vi "GUI_HTU_Chicane.vi"() -> ()   [LabVIEW 2013]
uses:
  Shared/GUI_Template/GUI_master/tcp_new_data_event.ctl
  Shared/GUI_Template/GUI_master/tcp new data cluster.ctl
panel:
  in  "Voltage::1":dbl caption="Outer Voltage" min=0.0 max=15.0
  in  "Voltage::2":dbl caption="Inner Voltage" min=0.0 max=15.0
  in  "Enable_Output::2":enum16{"on", "off"}(ring) caption="Enable output inner"
  in  "Enable_Output::1":enum16{"on", "off"}(ring) caption="Enable output outer"
  in  "RunList::2":enum16{"on", "off"}(ring) caption="Run List Inner Pair"
  in  "RunList::1":enum16{"on", "off"}(ring) caption="Run List Outer Pair"
  in  "LoadList::2":enum16{"on", "off"}(ring) caption="Load List Inner Pair"
  in  "LoadList::1":enum16{"on", "off"}(ring) caption="Load List Outer Pair"
  out "Chart":dbl[][](graph)
  in  "ApplyChicaneSettings":bool
  in  "Energy (MeV)":dbl=100.0
  in  "R56 (microns)":dbl
  out "Offset (mm)":dbl
  out "Width of 2% \nenergy spread (mm)":dbl
  out "SetCurrent":dbl
  in  "CalculateChicaneSettings":bool
  in  "Current::1":dbl caption="Outer Current" min=-12.0 max=12.0
  in  "Current::2":dbl caption="Inner Current" min=-12.0 max=12.0
  out "error IO 2":errorcluster
  out "tcp data event":T1
  in  "UDP error message":string
  in  "GUIdevice 2":string="U_ChicaneInner"
  in  "GUIdevice 1":string="U_ChicaneOuter"
  in  "stop":bool
  # "HTU Chicane"
  # "Energy"
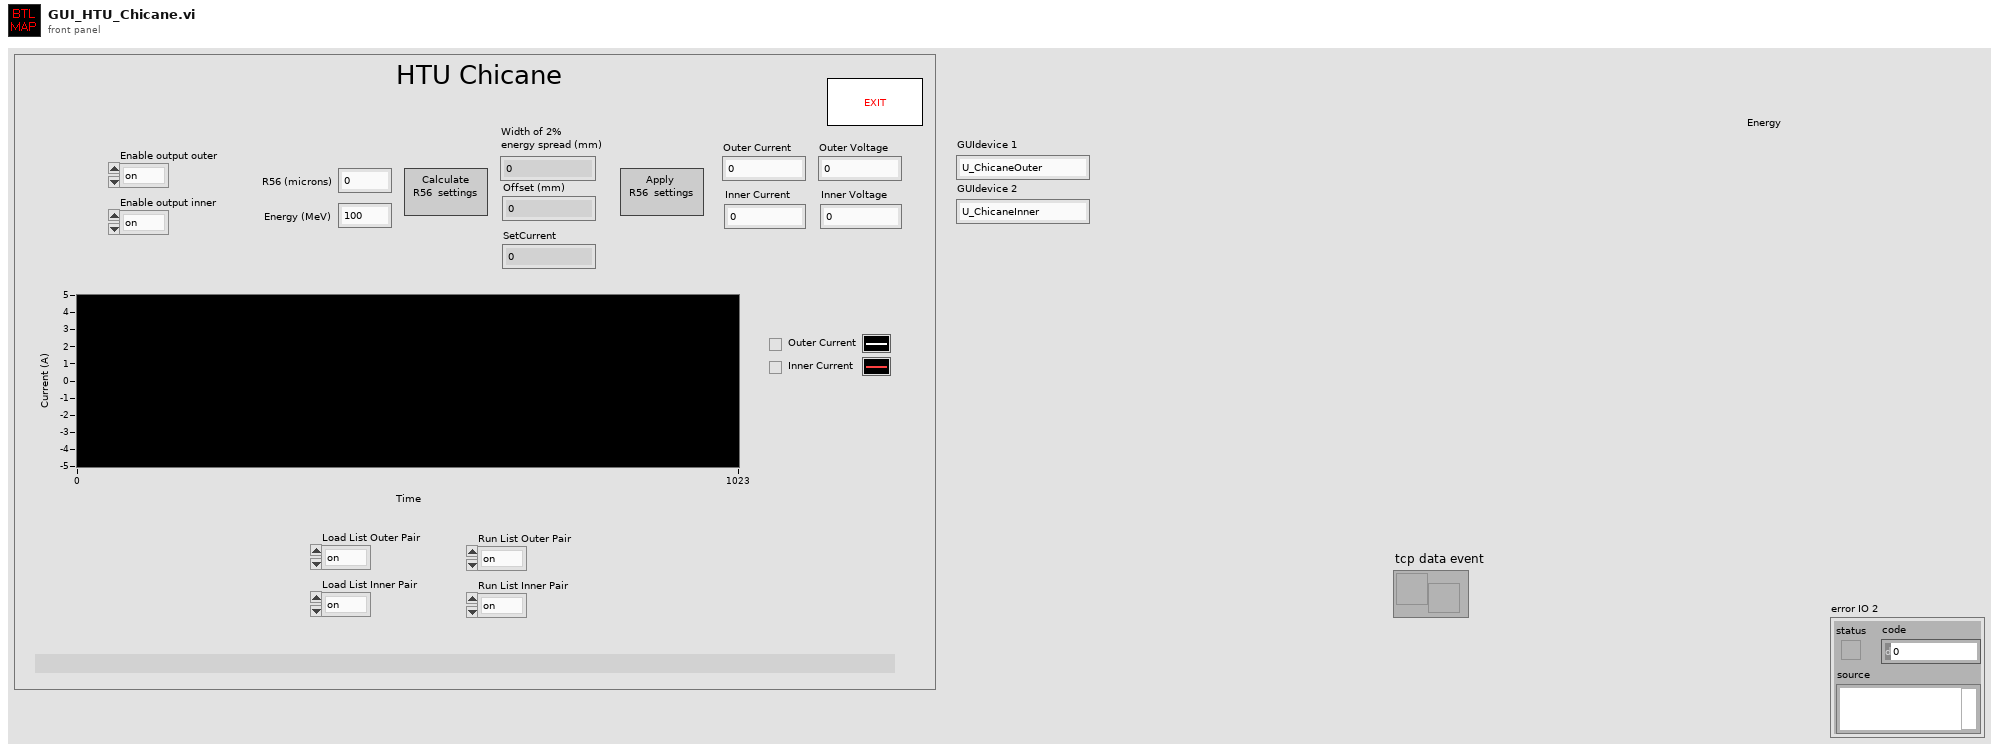
[diagram p1: front panel]
types:
  T1 = typedef "tcp_new_data_event.ctl" = refnum<user-event>
  T2 = typedef "tcp new data cluster.ctl" = cluster{"EventEnum":enum16{"new data", "connection status update"}, "Device name":string}
  T3 = enum32{"invalid app kind", "Development System", "Run Time System", "Student Edition", "Embedded LabVIEW", "Evaluation", "Custom"}
  T4 = enum32{"Invalid", "Standard", "Closed", "Hidden", "Minimized", "Maximized"}
  T5 = cluster{"Core":cluster{"Current VI Reference":refnum<vi>, "Close Panel on Exit?":bool}, "CalculateChicanceSettings":bool, "ApplyChicanceSettings":bool, "CurrentGraph1":dbl[][], "CurrentGraph2":dbl[][]}
  T6 = cluster{"Current VI Reference":refnum<vi>, "Close Panel on Exit?":bool}
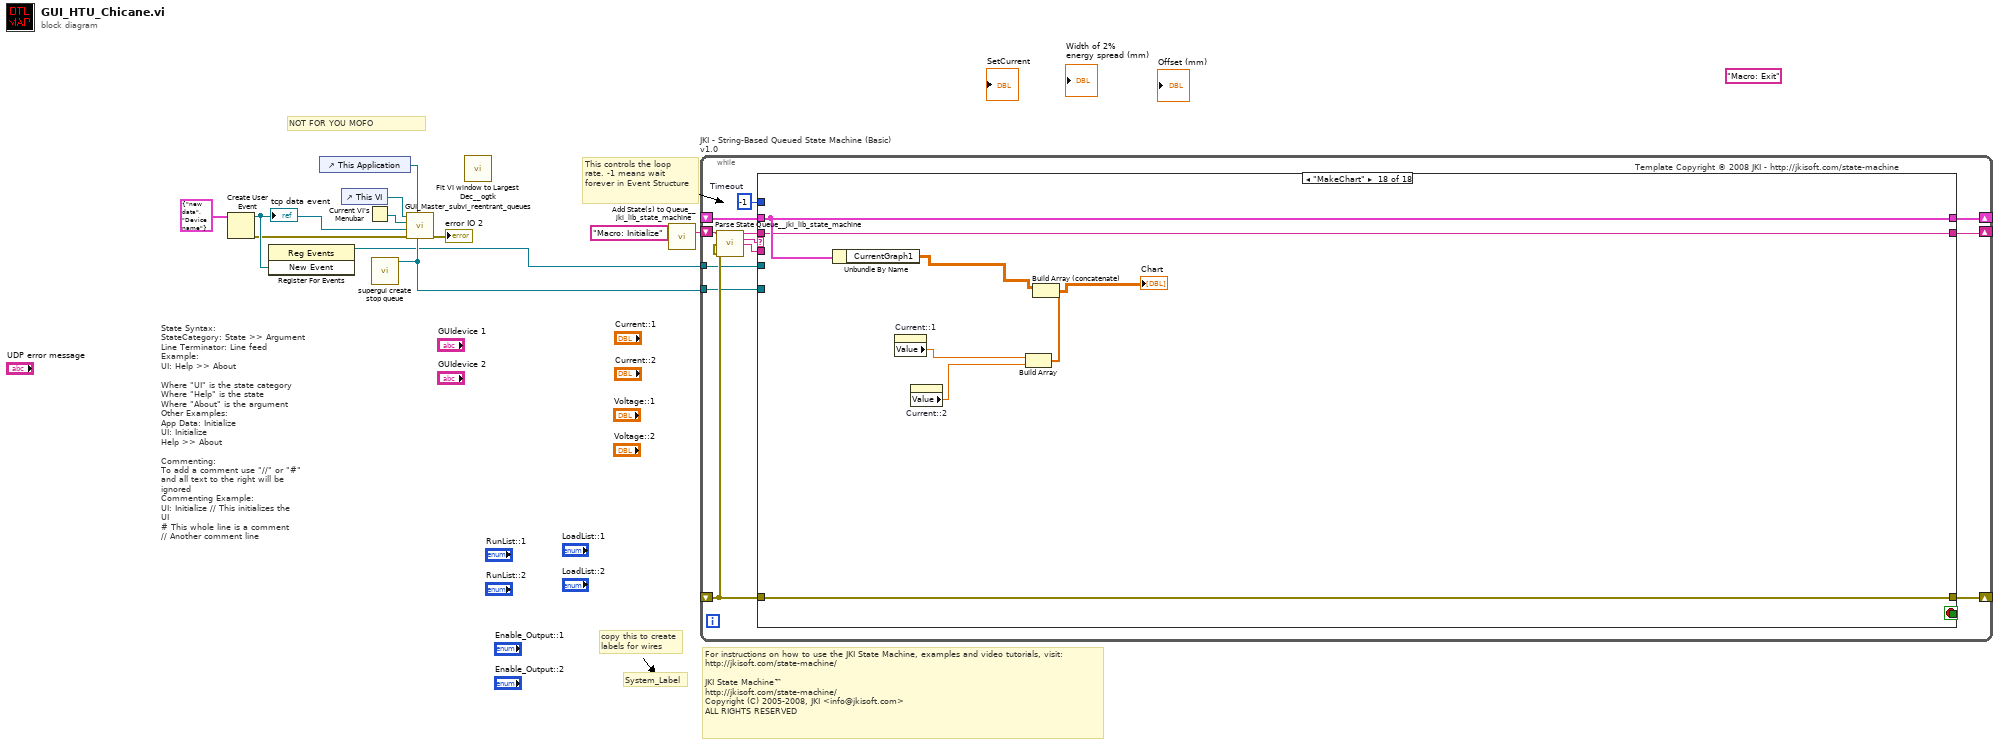
[diagram p0: block diagram]
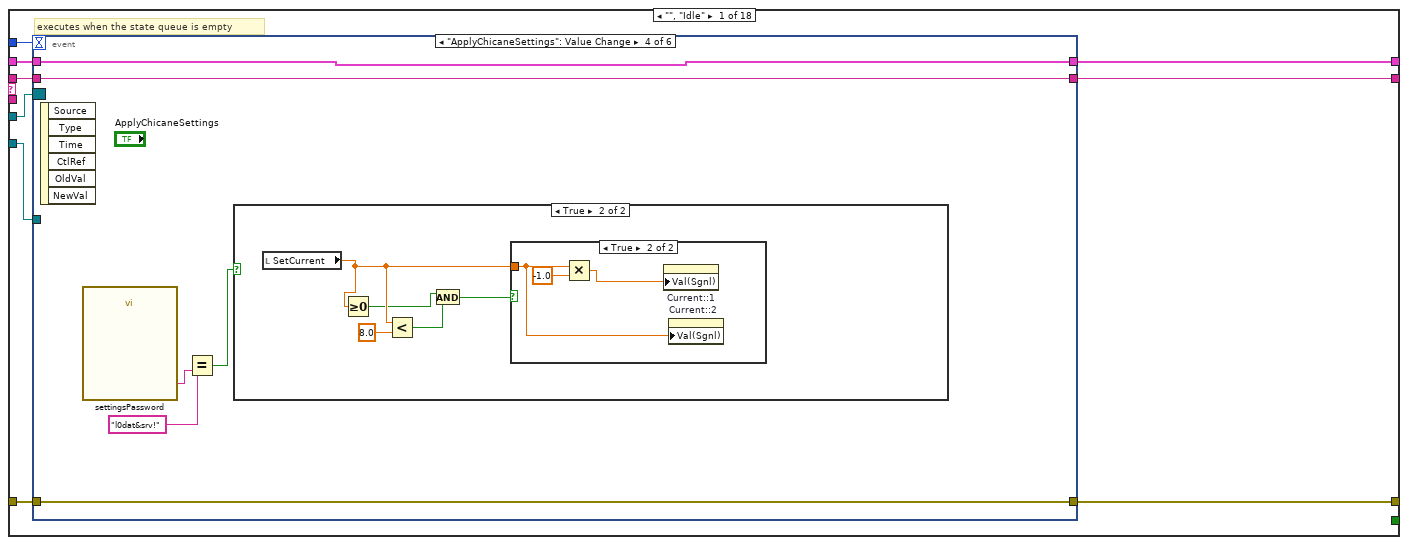
[diagram p2: hidden frame]
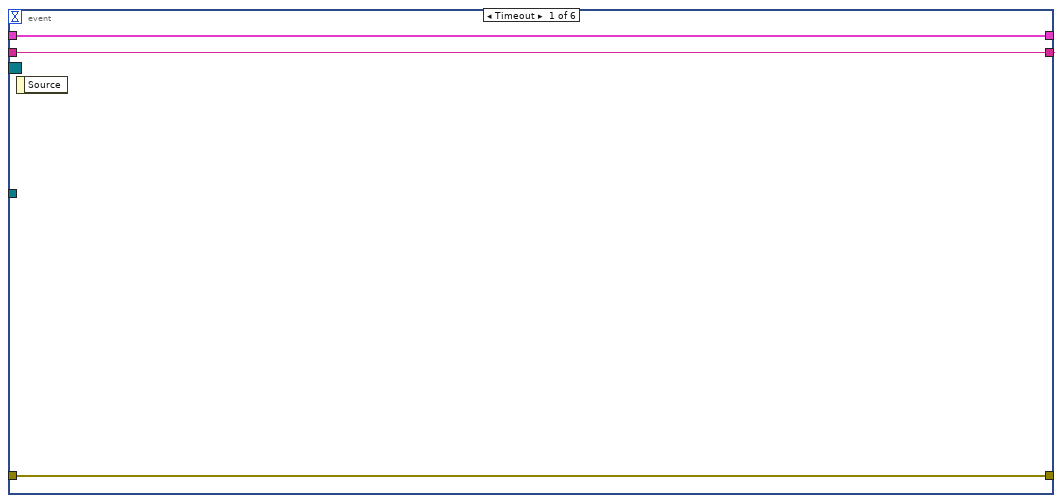
[diagram p3: hidden frame]
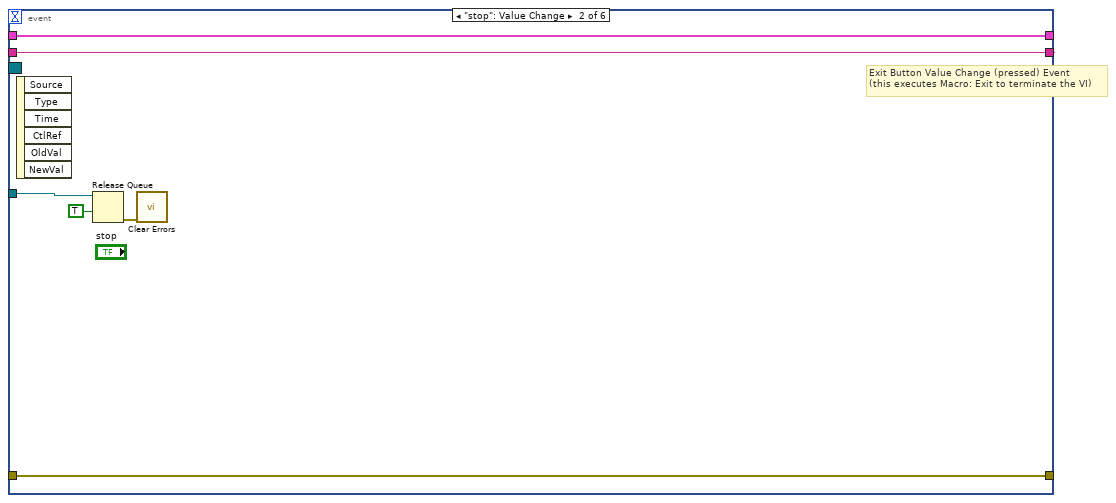
[diagram p4: hidden frame]
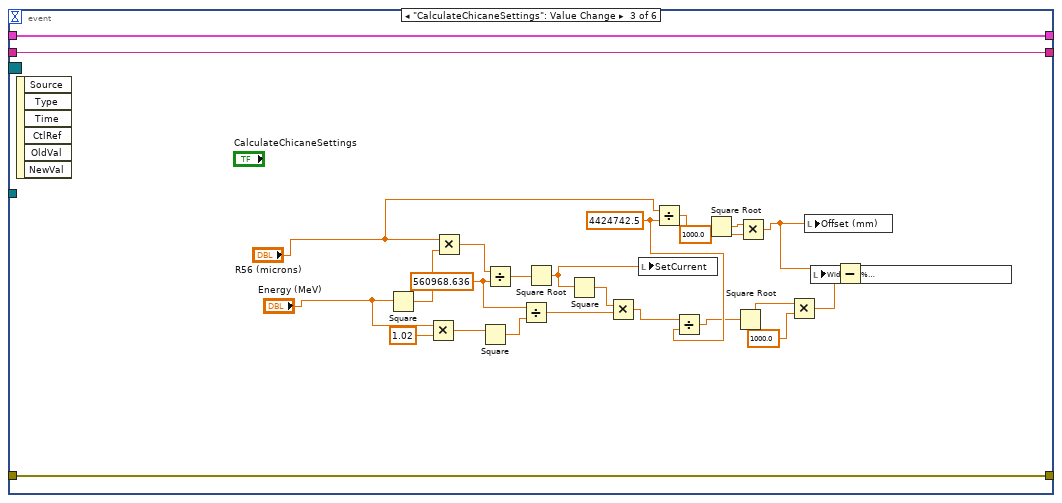
[diagram p5: hidden frame]
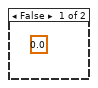
[diagram p6: hidden frame]
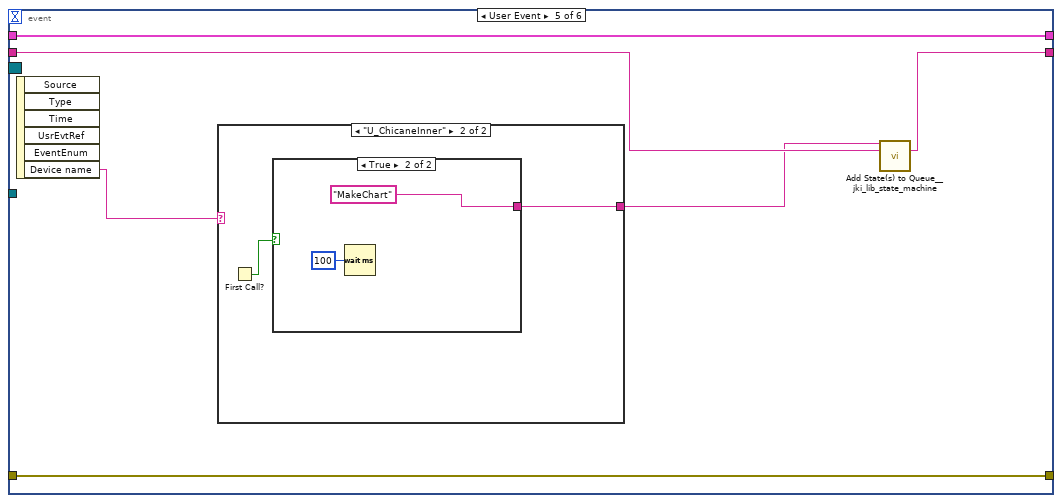
[diagram p8: hidden frame]
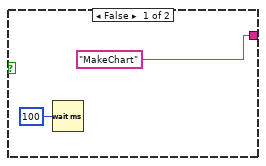
[diagram p10: hidden frame]
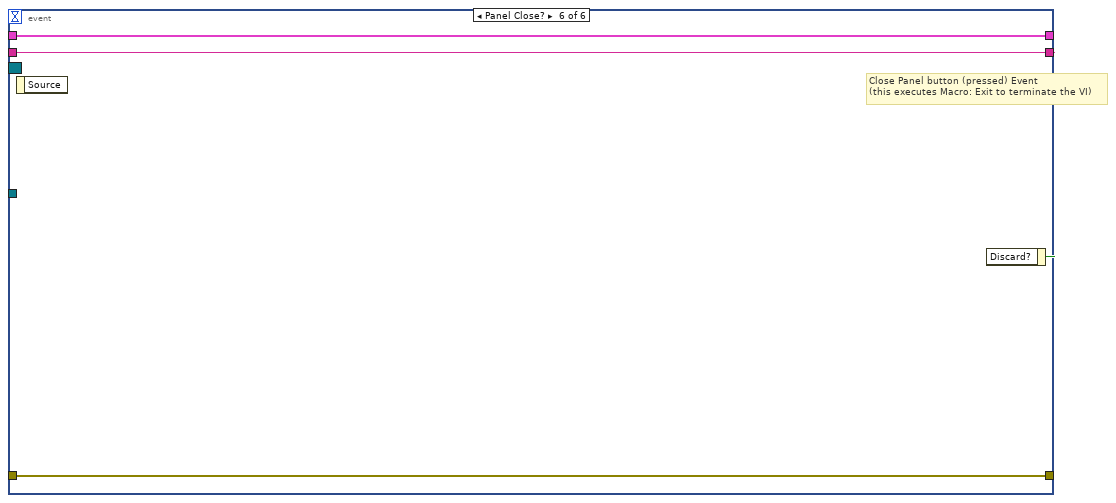
[diagram p11: hidden frame]
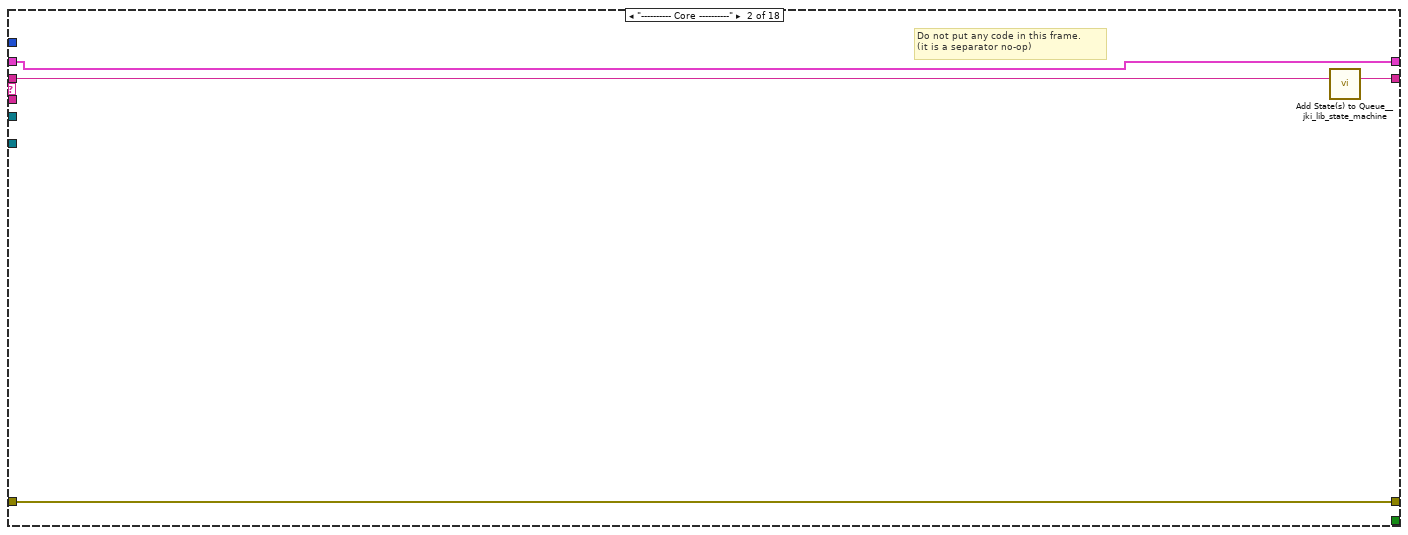
[diagram p12: hidden frame]
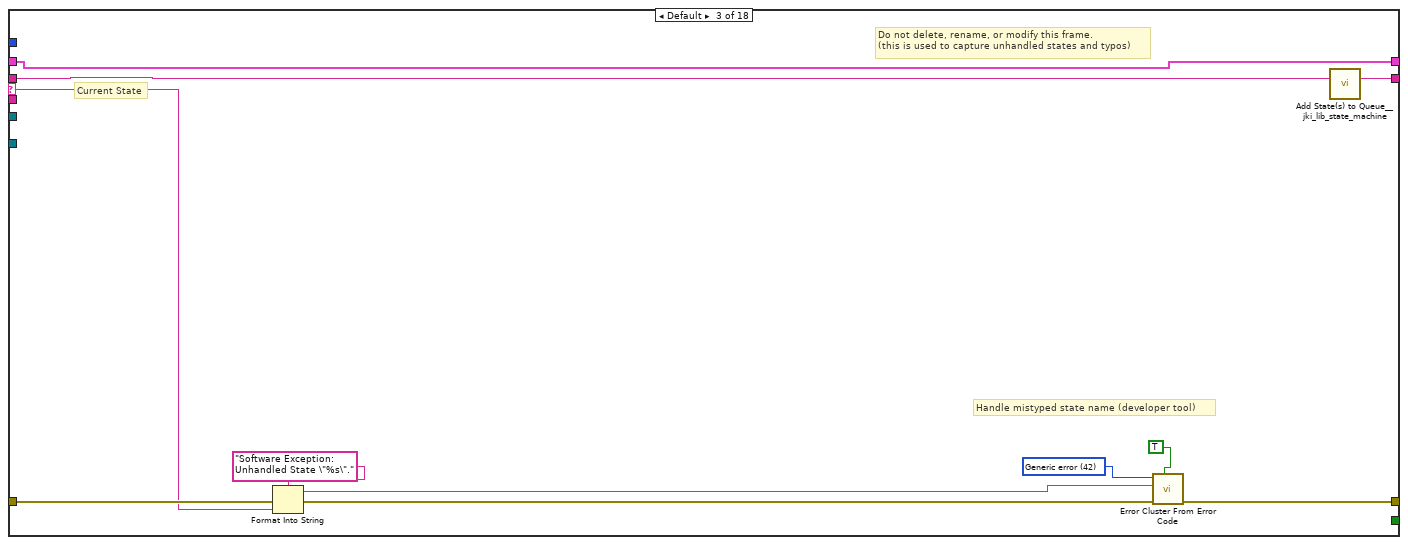
[diagram p13: hidden frame]
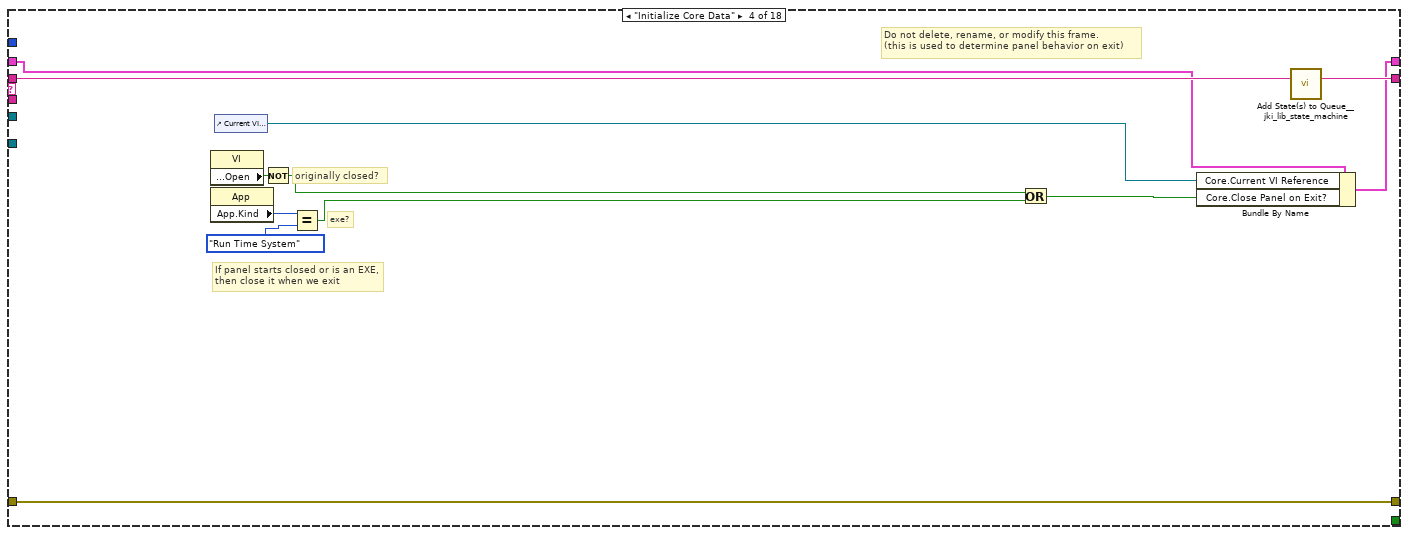
[diagram p14: hidden frame]
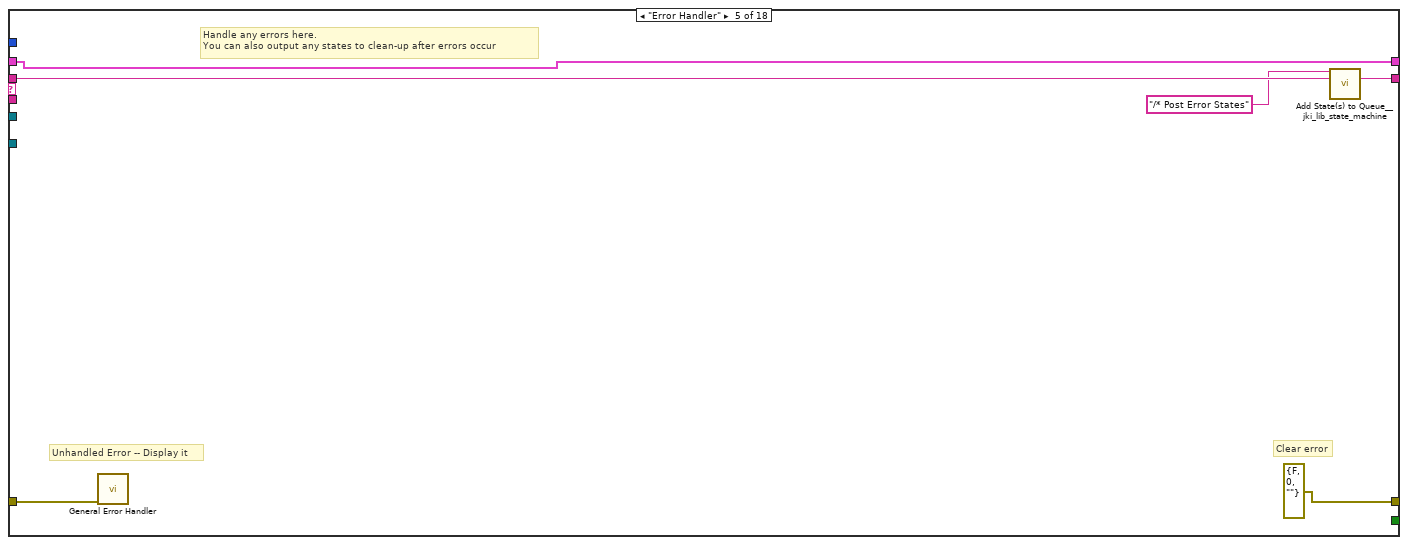
[diagram p15: hidden frame]
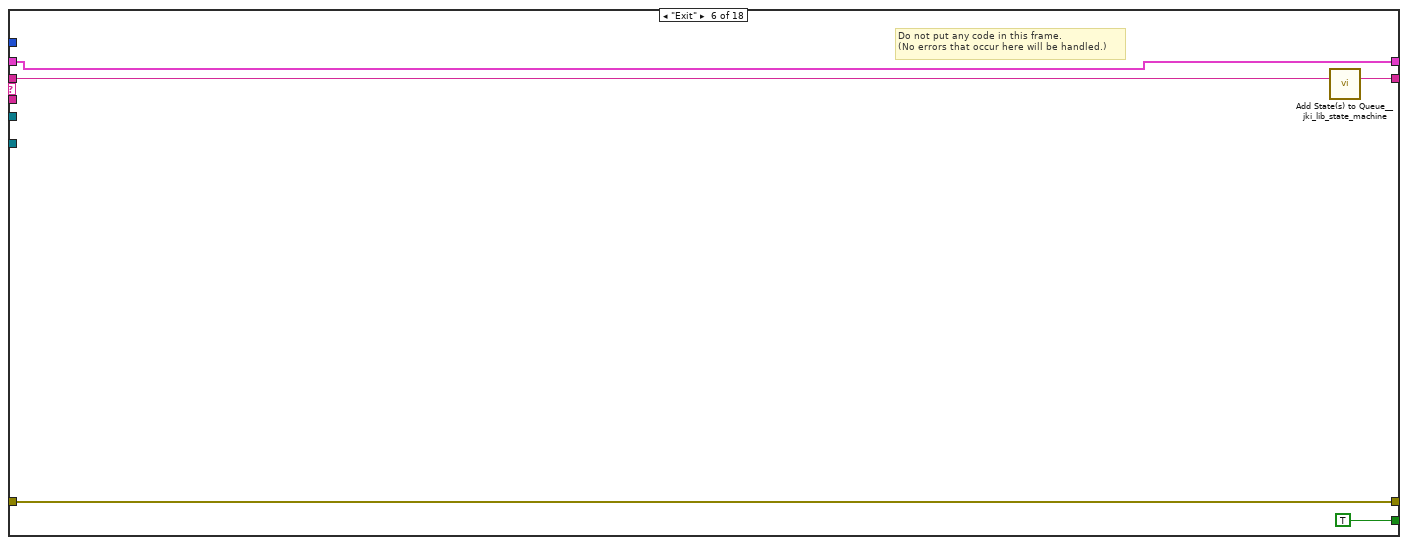
[diagram p16: hidden frame]
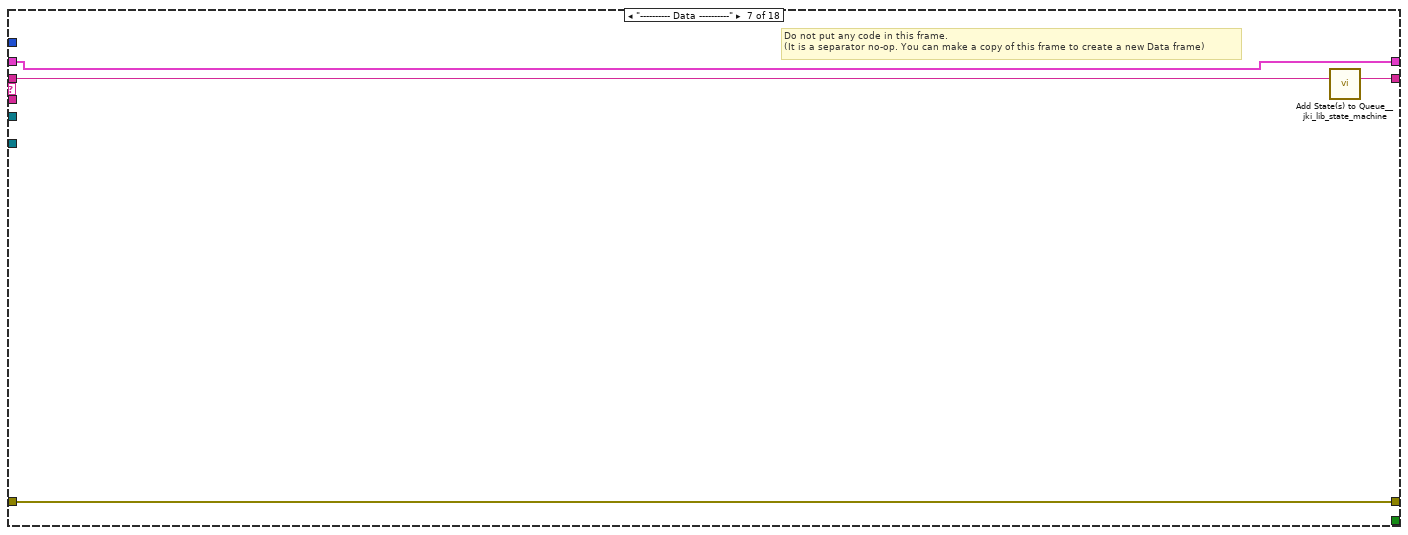
[diagram p17: hidden frame]
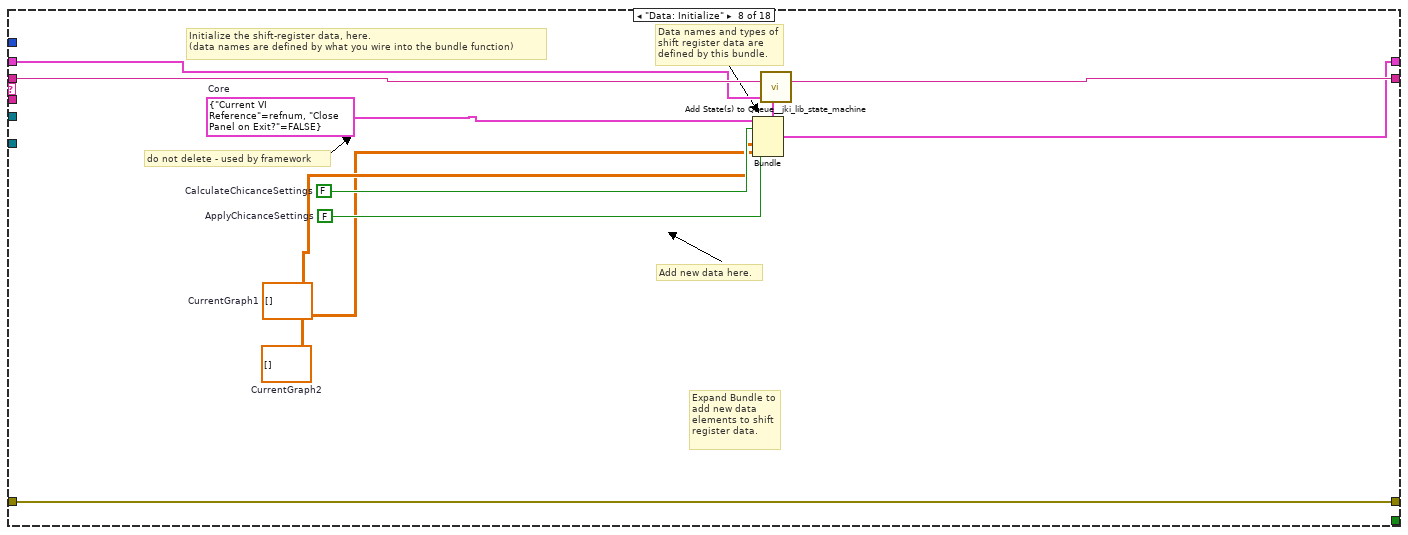
[diagram p18: hidden frame]
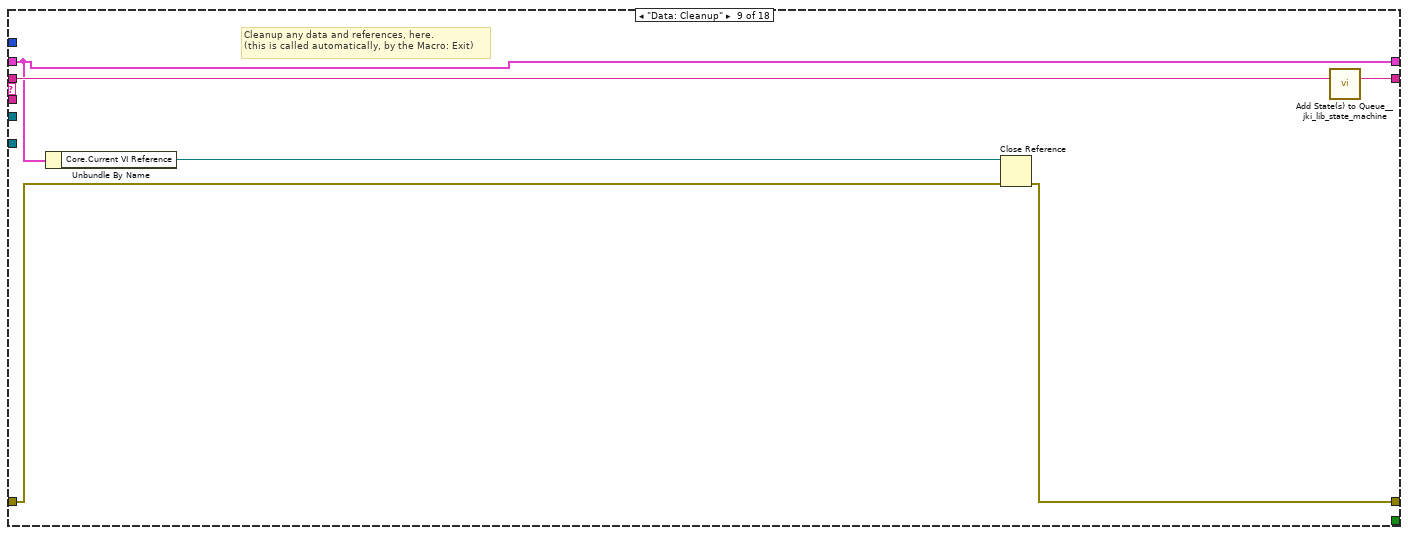
[diagram p19: hidden frame]
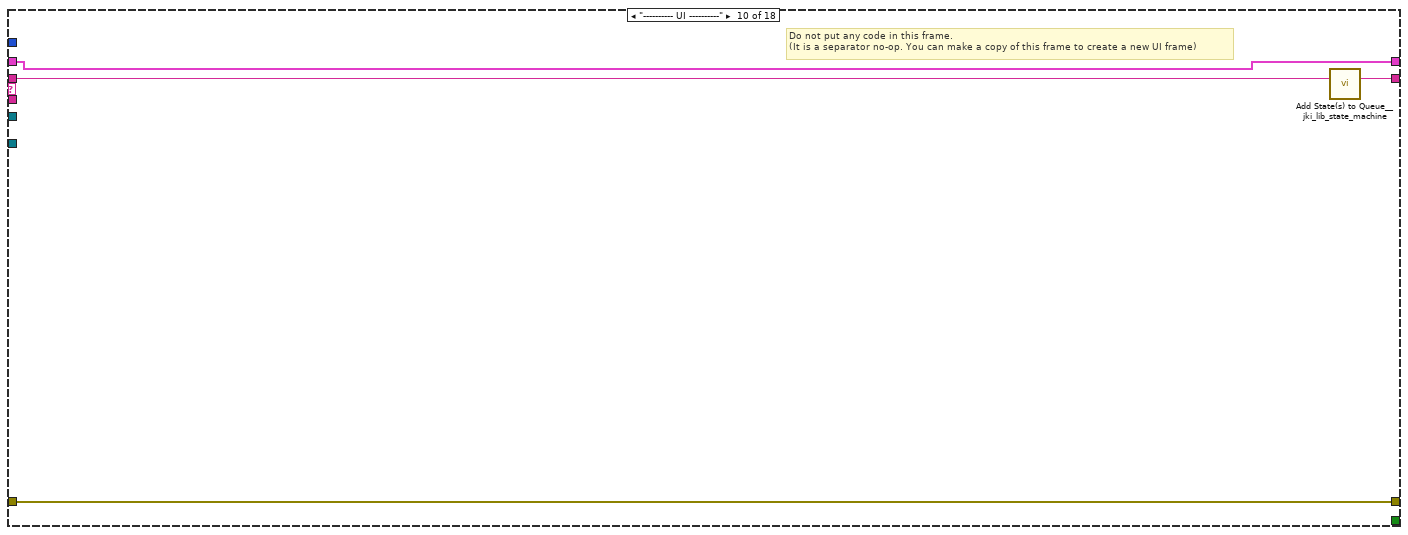
[diagram p20: hidden frame]
diagram:
  (unwired) "Macro: Exit"
  # "For instructions on how to use the JKI State Machine, examples and video tutorials, visit:\nhttp://jkisoft.com/state-machine/\n\nJKI State Machine™\nhttp://jkisoft.com/state-machine/\nCopyright (C) 2005-2008, JKI <info@jkisoft.com>\nALL RIGHTS RESERVED"
  # "State Syntax:\nStateCategory: State >> Argument\nLine Terminator: Line feed\nExample:\nUI: Help >> About\n\nWhere \"UI\" is the state category\nWhere \"Help\" is the state\nWhere \"About\" is the argument\nOther Examples:\nApp Data: Initialize\nUI: Initialize\nHelp >> About\n\nCommenting:\nTo add a comment use \"//\" or \"#\" and all text to the right will be ignored\nCommenting Example:\nUI: Initialize // This initializes the UI\n# This whole line is a comment\n// Another comment line"
  # "copy this to create labels for wires"
  # "This controls the loop rate. -1 means wait forever in Event Structure"
  # "System_Label"
  # "NOT FOR YOU MOFO"
  n1 = Create User Event(user event datatype=T2 {"EventEnum"=enum."new data", "Device name"="Device name"} ("New Event")) -> (user event=w10:refnum<user-event>, error out=w9:errorcluster)  [unwired: 1 in]
  "tcp data event" <- w10
  n2 = register-events(w10) -> (reference out=w1:refnum<event-registration>)  [unwired: 2 in, 1 out]
  n3 = control-ref of="This Application"() -> (w11:refnum<vi>)
  n4 = control-ref of="This VI"() -> (w5:refnum<vi>)
  n5 = Current VI's Menubar() -> (w7:refnum<k9>)
  n6 = call "supergui create stop queue.vi"() -> ("STOP Queue out"=w2:refnum<queue>)  [unwired: 11 in]
  n7 = call "GUI_Master_subvi_reentrant_queues.vi"("STOP Queue in"=w2, "This Application"=w11, "error in (no error)"=w9, "tcp data event"=w10, "Caller menu reference"=w7, "Caller VI ref"=w5) -> ("error out"=→"error IO 2":errorcluster)  [unwired: 5 in]
  n8 = call <userlib>:"Fit VI window to Largest Dec__ogtk.vi"() -> ()  [unwired: 6 in, 2 out]
  n9 = call <vilib>:"Add State(s) to Queue__jki_lib_state_machine.vi"("State(s) in (\"\")"="Macro: Initialize") -> ("States Out"=w3:string)  [unwired: 14 in]
  n10 = while "JKI - String-Based Queued State Machine (Basic) v1.0" {
    shift-right: [w17] -> _
    shift-left: _ -> [w16]
    shift-right: [w20] -> _
    shift-left: _ -> [w14]
    shift-right: [w19] -> _
    shift-left: w3 -> [w21]
    tunnel: w1 -> [w13]
    tunnel: w2 -> [w12]
    stop <- w18 stop-if-true
    w15 = -1  # Timeout
    # "Template Copyright © 2008 JKI - http://jkisoft.com/state-machine"
    n11 = call <vilib>:"Parse State Queue__jki_lib_state_machine.vi"("State Queue"=w21, "Error In (no error)"=w14) -> ("Remaining States"=w23:string, "Current State"=w24:string, "Arguments"=w22:string)  [unwired: 11 in]
    n12 = case shown="\"MakeChart\"" w24 {
      selector: w24 -> [_ _ w108 _ _ _ _ _ _ _ _ _ _ _ _ _ _ _]
      tunnel: w23 -> [w33 w107 w112 w130 w136 w141 w145 w155 w161 w165 w169 w175 w186 w212 w217 w227 w231 w236]
      tunnel: w22 -> [_ _ _ _ _ _ _ _ _ _ _ w170 w181 _ _ _ _ _]
      tunnel: w16 -> [w31 w104 w110 w120 w133 w139 w142 w150 w156 w162 w167 w173 w180 w209 w214 w218 w228 w237]
      tunnel: [w30 w105 w114 w128 errorcluster {"status"=FALSE, "code"=0, "source"=""} ("error out") w138 w143 w153 w158 w163 w166 w171 w183 w210 w215 w225 w229 w235] -> w20
      tunnel: w14 -> [w29 w105 w113 w128 w132 w138 w143 w153 w159 w163 w166 w172 w184 w210 w215 w225 w229 w235]
      tunnel: [w32 w106 w111 w129 w135 w140 w144 w154 w160 w164 w168 w174 w185 w211 w216 w226 w230 w236] -> w19
      tunnel: [_ _ _ _ _ TRUE _ _ _ _ _ _ _ _ _ _ _ _] -> w18
      tunnel: [w25 w104 w110 w119 w133 w139 w142 w149 w156 w162 w167 w173 w180 w209 w214 w218 w228 w237] -> w17
      tunnel: w15 -> [w28 _ _ _ _ _ _ _ _ _ _ _ _ _ _ _ _ _]
      tunnel: w13 -> [w27 _ _ _ _ _ _ _ _ _ _ _ _ _ _ _ _ _]
      tunnel: w12 -> [w26 _ _ _ _ _ _ _ _ _ _ _ _ _ _ _ _ _]
      frame "", "Idle" {
        # "executes when the state queue is empty"
        n13 = event shown="[3] \"ApplyChicaneSettings\": Value Change" {
          selector: w27 -> [_ _ _ _ _ _]
          dyn-events: _ -> [_ _ _ _ _ _]
          timeout: w28 -> [_ _ _ _ _ _]
          tunnel: w33 -> [w37 w45 w71 w77 w89 w103]
          tunnel: [w36 w44 w71 w77 w87 w102] -> w32
          tunnel: w31 -> [w34 w42 w69 w73 w90 w100]
          tunnel: [w35 w43 w70 w76 w86 w101] -> w30
          tunnel: w29 -> [w35 w43 w70 w76 w86 w101]
          tunnel: [w34 w42 w69 w73 w90 w100] -> w25
          tunnel: w26 -> [_ w39 _ _ _ _]
          event Timeout {
            n14 = event-data() -> ()  [unwired: 1 in, 1 out]
            n15 = call <vilib>:"Add State(s) to Queue__jki_lib_state_machine.vi"("State(s) in (\"\")"=w37) -> ("States Out"=w36:string)  [unwired: 14 in]
          }
          event "stop": Value Change {
            # "Exit Button Value Change (pressed) Event\n(this executes Macro: Exit to terminate the VI)"
            n16 = event-data() -> ()  [unwired: 1 in, 6 out]
            n17 = Release Queue(queue=w39, force destroy? (F)=TRUE) -> (error out=w40:errorcluster)  [unwired: 1 in, 2 out]
            n18 = call <vilib>:"Clear Errors.vi"("error in (no error)"=w40) -> ()  [unwired: 6 in, 1 out]
            n19 = call <vilib>:"Add State(s) to Queue__jki_lib_state_machine.vi"("State(s) in Front (\"\")"="Macro: Exit", "State(s) in (\"\")"=w45) -> ("States Out"=w44:string)  [unwired: 13 in]
          }
          event "CalculateChicaneSettings": Value Change {
            w52 = 4424742.5 ("y")
            w59 = 560968.636 ("y")
            n20 = event-data() -> ()  [unwired: 1 in, 6 out]
            n21 = Square(x="Energy (MeV)") -> (x^2=w54:dbl)
            n22 = Multiply(x="Energy (MeV)", y=1.02) -> (x*y=w58:dbl)
            n23 = Multiply(x="R56 (microns)", y=w54) -> (x*y=w55:dbl)
            n24 = Square(x=w58) -> (x^2=w60:dbl)
            n25 = Divide(x=w55, y=w59) -> (x/y=w64:dbl)
            n26 = Divide(x=w59, y=w60) -> (x/y=w61:dbl)
            n27 = Square Root(x=w64) -> (sqrt(x)=w65:dbl)
            n28 = Square(x=w65) -> (x^2=w62:dbl)
            n29 = Multiply(x=w62, y=w61) -> (x*y=w53:dbl)
            n30 = local write "SetCurrent"(w65) -> ()
            n31 = Divide(x="R56 (microns)", y=w52) -> (x/y=w66:dbl)
            n32 = Divide(x=w53, y=w52) -> (x/y=w51:dbl)
            n33 = Square Root(x=w66) -> (sqrt(x)=w68:dbl)
            n34 = Square Root(x=w51) -> (sqrt(x)=w50:dbl)
            n35 = Multiply(x=w68, y=1000.0) -> (x*y=w48:dbl)
            n36 = Multiply(x=w50, y=1000.0) -> (x*y=w47:dbl)
            n37 = local write "Offset (mm)"(w48) -> ()
            n38 = Subtract(x=w48, y=w47) -> (x-y=w46:dbl)
            n39 = local write "Width of 2% \nenergy spread (mm)"(w46) -> ()
          }
          event "ApplyChicaneSettings": Value Change {
            n40 = event-data() -> ()  [unwired: 1 in, 6 out]
            n41 = call "settingsPassword.vi"() -> ("password"=w75:string)  [unwired: 17 in, 2 out]
            n42 = Equal?(x="l0dat&srv!", y=w75) -> (x = y?=w72:bool)
            n43 = case shown="True" w72 {
              frame False {
                (unwired) 0.0 ("opening Time")
              }
              frame True {
                n44 = local read "SetCurrent"() -> (w82:dbl)
                n45 = Greater Or Equal To 0?(x=w82) -> (x >= 0?=w80:bool)
                n46 = Less?(x=w82, y=8.0) -> (x < y?=w79:bool)
                n47 = And(x=w80, y=w79) -> (x .and. y?=w78:bool)
                n48 = case shown="True" w78 {
                  tunnel: w82 -> [_ w83]
                  frame False {
                  }
                  frame True {
                    n49 = Multiply(x=w83, y=-1.0) -> (x*y=w84:dbl)
                    n50 = property on="Current::1" class="DigNum (strict)"("Val(Sgnl)"=w84) -> ()  [unwired: 2 in, 2 out]
                    n51 = property on="Current::2" class="DigNum (strict)"("Val(Sgnl)"=w83) -> ()  [unwired: 2 in, 2 out]
                  }
                }
              }
            }
          }
          event User Event {
            n52 = event-data() -> ("Device name"=w91:string)  [unwired: 1 in, 5 out]
            n53 = case shown="\"U_ChicaneInner\"" w91 {
              tunnel: [_ w93] -> w88
              frame "False", Default {
              }
              frame "U_ChicaneInner" {
                n54 = First Call?() -> (First Call?: T/F=w92:bool)
                n55 = case shown="True" w92 {
                  tunnel: ["MakeChart" "MakeChart"] -> w93
                  frame False {
                    n56 = Wait (ms)(milliseconds to wait=u32 100) -> ()  [unwired: 1 out]
                  }
                  frame True {
                    n57 = Wait (ms)(milliseconds to wait=u32 100) -> ()  [unwired: 1 out]
                  }
                }
              }
            }
            n58 = call <vilib>:"Add State(s) to Queue__jki_lib_state_machine.vi"("State(s) in Front (\"\")"=w88, "State(s) in (\"\")"=w89) -> ("States Out"=w87:string)  [unwired: 13 in]
          }
          event Panel Close? {
            # "Discard the event because we'll close the front panel ourselves in Macro: Exit"
            # "Close Panel button (pressed) Event\n(this executes Macro: Exit to terminate the VI)"
            n59 = event-data() -> ()  [unwired: 1 in, 1 out]
            n60 = event-data("Discard?"=TRUE) -> ()  [unwired: 1 in, 1 out]
            n61 = call <vilib>:"Add State(s) to Queue__jki_lib_state_machine.vi"("State(s) in Front (\"\")"="Macro: Exit", "State(s) in (\"\")"=w103) -> ("States Out"=w102:string)  [unwired: 13 in]
          }
        }
      }
      frame "---------- Core ----------" {
        # "Do not put any code in this frame.\n(it is a separator no-op)"
        n62 = call <vilib>:"Add State(s) to Queue__jki_lib_state_machine.vi"("State(s) in (\"\")"=w107) -> ("States Out"=w106:string)  [unwired: 14 in]
      }
      frame Default {
        w117 = 42 items=["No error", "Argument error", "Memory is full", "Out of zone", "End of file", "File already open", "Generic file I/O error", "File not found", "File permission error", "Disk is full", "Duplicate path", "Too many files open", "System feature not enabled", "Resource file not found", "Cannot add resource", "Resource not found", "Image not found", "Image memory error", "Pen does not exist", "Config type invalid", "Config token not found", "Config parse error", "Config memory error", "Bad external code format", "Bad external code offset", "External code not present", "Null window", "Destroy window error", "Null menu", "Print aborted", "Bad print record", "Print driver error", "Windows error during printing", "Memory error during printing", "Print dialog error", "Generic print error", "Invalid device refnum", "Device not found", "Device parameter error", "Device unit error", "Cannot open device", "Device call aborted", "Generic error", "Cancelled by user", "Object ID too low", "Object ID too high", "Object not in heap", "Unknown heap", "Unknown object (invalid DefProc)", "Unknown object (DefProc not in table)", "Message out of range", "Invalid (null) method", "Unknown message", "Manager call not supported", "Bad address", "Network operation in progress", "Network operation timed out", "Connection is busy", "Network attribute not supported", "Network error", "Address in use", "System out of memory", "Connection aborted", "Connection refused", "Not connected", "Already connected", "Connection closed", "Initialization error (interapplication manager)", "Bad occurrence", "Wait on unbound occurrence handler", "Occurrence queue overflow", "Datalog type conflict", "Unused", "Unrecognized type (interapplication manager)", "Memory corrupt", "Failed to make temporary DLL", "Old CIN version", "Drag socket not found", "Failed to load drop-object", "Failed to register OLE object", "Failed to release OLE object", "Format specifier type mismatch", "Unknown format specifier", "Too few format specifiers", "Too many format specifiers", "Scan failed", "Newer CIN version", "Error converting to variant", "Runtime menu error", "Password tampered", "Variant attribute not found", "Incompatible variant data type", "Event data is not available", "Event Store is not present", "Occurrence is not found", "Event Queue is not created", "Event info is not available", "Refnum passed is NULL", "Error retrieving Class GUID", "Error retrieving CoClass GUID", "Error retrieving TypeLib GUID.", "Bad built application magic bytes.", "Specific driver is different from the specific driver associated with the Logical Name.", "There is no session opened to the class driver.", "Max Error", "MAX - Error with config objects", "MAX - Error loading configuration", "MAX - Group not supported"]
        # "Current State"
        # "Do not delete, rename, or modify this frame.\n(this is used to capture unhandled states and typos)"
        # "Handle mistyped state name (developer tool)"
        n63 = Format Into String(format string="Software Exception: Unhandled State \"%s\"." ("message"), error in=w113, w108) -> (resulting string=w116:string, error out=w115:errorcluster)  [unwired: 1 in]
        n64 = call <vilib>:"Error Cluster From Error Code.vi"("show call chain? (False)"=TRUE, "error in (no error)"=w115, "error message (\"\")"=w116, "error code (0)"=w117) -> ("error out"=w114:errorcluster)  [unwired: 5 in]
        n65 = call <vilib>:"Add State(s) to Queue__jki_lib_state_machine.vi"("State(s) in (\"\")"=w112) -> ("States Out"=w111:string)  [unwired: 14 in]
      }
      frame "Initialize Core Data" {
        # "Do not delete, rename, or modify this frame.\n(this is used to determine panel behavior on exit)"
        # "originally closed?"
        # "exe?"
        # "If panel starts closed or is an EXE, then close it when we exit"
        n66 = property class="VI"() -> ("Front Panel.Open"=w127:bool)  [unwired: 2 in, 2 out]
        n67 = property class="App"() -> ("App.Kind"=w126:T3)  [unwired: 2 in, 2 out]
        n68 = control-ref of="Current VI Reference"() -> (w121:refnum<vi>)
        n69 = Not(x=w127) -> (.not. x?=w124:bool)
        n70 = Equal?(x=w126, y=T3."Run Time System" ("Application:Kind")) -> (x = y?=w123:bool)
        n71 = Or(x=w124, y=w123) -> (x .or. y?=w122:bool)
        n72 = Bundle By Name(cluster=w120, "Core.Current VI Reference"=w121, "Core.Close Panel on Exit?"=w122) -> (w119:T5)
        n73 = call <vilib>:"Add State(s) to Queue__jki_lib_state_machine.vi"("State(s) in (\"\")"=w130) -> ("States Out"=w129:string)  [unwired: 14 in]
      }
      frame "Error Handler" {
        # "Unhandled Error -- Display it"
        # "Handle any errors here.\nYou can also output any states to clean-up after errors occur"
        # "Clear error"
        n74 = call <vilib>:"General Error Handler.vi"("error in (no error)"=w132) -> ()  [unwired: 10 in, 5 out]
        n75 = call <vilib>:"Add State(s) to Queue__jki_lib_state_machine.vi"("State(s) in Front (\"\")"="/* Post Error States", "State(s) in (\"\")"=w136) -> ("States Out"=w135:string)  [unwired: 13 in]
      }
      frame "Exit" {
        # "Do not put any code in this frame.\n(No errors that occur here will be handled.)"
        n76 = call <vilib>:"Add State(s) to Queue__jki_lib_state_machine.vi"("State(s) in (\"\")"=w141) -> ("States Out"=w140:string)  [unwired: 14 in]
      }
      frame "---------- Data ----------" {
        # "Do not put any code in this frame.\n(It is a separator no-op. You can make a copy of this frame to create a new Data frame)"
        n77 = call <vilib>:"Add State(s) to Queue__jki_lib_state_machine.vi"("State(s) in (\"\")"=w145) -> ("States Out"=w144:string)  [unwired: 14 in]
      }
      frame "Data: Initialize" {
        w146 = dbl[][] []  # CurrentGraph2
        w147 = dbl[][] []  # CurrentGraph1
        w148 = FALSE  # ApplyChicanceSettings
        w151 = FALSE  # CalculateChicanceSettings
        w152 = T6 {"Current VI Reference"=refnum, "Close Panel on Exit?"=FALSE}  # Core
        # "do not delete - used by framework"
        # "Expand Bundle to add new data elements to shift register data."
        # "Add new data here."
        # "Data names and types of shift register data are defined by this bundle."
        # "Initialize the shift-register data, here.\n(data names are defined by what you wire into the bundle function)"
        n78 = Bundle(cluster=w150, "Core"=w152, "CalculateChicanceSettings"=w151, "ApplyChicanceSettings"=w148, "CurrentGraph1"=w147, "CurrentGraph2"=w146) -> (w149:T5)
        n79 = call <vilib>:"Add State(s) to Queue__jki_lib_state_machine.vi"("State(s) in (\"\")"=w155) -> ("States Out"=w154:string)  [unwired: 14 in]
      }
      frame "Data: Cleanup" {
        # "Cleanup any data and references, here.\n(this is called automatically, by the Macro: Exit)"
        n80 = Unbundle By Name(w156) -> ("Core.Current VI Reference"=w157:refnum<vi>)
        n81 = Close Reference(reference=w157, error in (no error)=w159) -> (error out=w158:errorcluster)
        n82 = call <vilib>:"Add State(s) to Queue__jki_lib_state_machine.vi"("State(s) in (\"\")"=w161) -> ("States Out"=w160:string)  [unwired: 14 in]
      }
      frame "---------- UI ----------" {
        # "Do not put any code in this frame.\n(It is a separator no-op. You can make a copy of this frame to create a new UI frame)"
        n83 = call <vilib>:"Add State(s) to Queue__jki_lib_state_machine.vi"("State(s) in (\"\")"=w165) -> ("States Out"=w164:string)  [unwired: 14 in]
      }
      frame "UI: Initialize" {
        # "Initialize the User Interface, here.\n(this is called automatically, by the Macro: Init)"
        n84 = call <vilib>:"Add State(s) to Queue__jki_lib_state_machine.vi"("State(s) in (\"\")"=w169) -> ("States Out"=w168:string)  [unwired: 14 in]
      }
      frame "UI: Cursor Set" {
        # "Argument"
        # "Set and Unset Cursor Busy.\n(Usage: \"UI: Cursor Set >> Busy|Idle\")"
        n85 = case shown="\"Idle\", Default" w170 {
          tunnel: w172 -> [w177 w179]
          tunnel: [w176 w178] -> w171
          frame "Idle", Default {
            n86 = call <vilib>:"Unset Busy.vi"("error in (no error)"=w177) -> ("error out"=w176:errorcluster)  [unwired: 10 in]
          }
          frame "Busy" {
            n87 = call <vilib>:"Set Busy.vi"("error in (no error)"=w179) -> ("error out"=w178:errorcluster)  [unwired: 9 in, 1 out]
          }
        }
        n88 = call <vilib>:"Add State(s) to Queue__jki_lib_state_machine.vi"("State(s) in (\"\")"=w175) -> ("States Out"=w174:string)  [unwired: 14 in]
      }
      frame "UI: Front Panel State" {
        # "Argument"
        # "Set Front Panel Open or Closed\n(Usage: \"UI: Front Panel State >> Open|Close\")"
        n89 = Unbundle By Name(w180) -> ("Core.Current VI Reference"=w182:refnum<vi>)
        n90 = case shown="\"Open\", Default" w181 {
          tunnel: w184 -> [w191 w203]
          tunnel: [w192 w204] -> w183
          tunnel: w182 -> [w187 w199]
          frame "Open", Default {
            n91 = property class="VI"(reference=w187, error in=w191) -> (reference out=w189:refnum<vi>, error out=w190:errorcluster, "Front Panel.Open"=w188:bool)
            n92 = case shown="False" w188 {
              tunnel: [w195 w198] -> w192
              tunnel: w190 -> [w194 w198]
              tunnel: w189 -> [w193 _]
              frame False {
                n93 = invoke class="VI" method="FP.Open"(reference=w193, error in=w194, "Activate"=TRUE, "State"=T4."Standard") -> (error out=w195:errorcluster)  [unwired: 1 in, 4 out]
              }
              frame True {
              }
            }
          }
          frame "Close" {
            n94 = property class="VI"(reference=w199, error in=w203) -> (reference out=w201:refnum<vi>, error out=w202:errorcluster, "Front Panel.Open"=w200:bool)
            n95 = case shown="True" w200 {
              tunnel: [w205 w208] -> w204
              tunnel: w202 -> [w205 w207]
              tunnel: w201 -> [_ w206]
              frame False {
              }
              frame True {
                n96 = invoke class="VI" method="FP.Close"(reference=w206, error in=w207) -> (error out=w208:errorcluster)  [unwired: 1 in, 2 out]
              }
            }
          }
        }
        n97 = call <vilib>:"Add State(s) to Queue__jki_lib_state_machine.vi"("State(s) in (\"\")"=w186) -> ("States Out"=w185:string)  [unwired: 14 in]
      }
      frame "---------- Macro ----------" {
        # "Do not put any code in this frame.\n(It is a separator no-op. You can make a copy of this frame to create a new Macro frame)"
        n98 = call <vilib>:"Add State(s) to Queue__jki_lib_state_machine.vi"("State(s) in (\"\")"=w212) -> ("States Out"=w211:string)  [unwired: 14 in]
      }
      frame "Macro: Initialize" {
        w213 = "Data: Initialize\nInitialize Core Data\nUI: Initialize\nUI: Front Panel State >> Open"  # Data: Initialize Initialize Core Data UI: Initialize UI: Front Panel State >> Open
        # "Initialization Macro\n(This is called once, when the VI starts)"
        n99 = call <vilib>:"Add State(s) to Queue__jki_lib_state_machine.vi"("State(s) in Front (\"\")"=w213, "State(s) in (\"\")"=w217) -> ("States Out"=w216:string)  [unwired: 13 in]
      }
      frame "Macro: Exit" {
        # "Exit Macro\n(This is called once, when the VI exits)"
        n100 = Unbundle By Name(w218) -> ("Core.Close Panel on Exit?"=w219:bool)
        n101 = Select(t="UI: Front Panel State >> Close", s=w219, f="") -> (s? t:f=w222:string)
        n102 = call <vilib>:"Add State(s) to Queue__jki_lib_state_machine.vi"("State(s) in (\"\")"=w222, "State(s) at Back (\"\")"="Data: Cleanup\nExit") -> ("States Out"=w220:string)  [unwired: 13 in]
        n103 = call <vilib>:"Add State(s) to Queue__jki_lib_state_machine.vi"("State(s) in Front (\"\")"=w220, "State(s) in (\"\")"=w227) -> ("States Out"=w226:string)  [unwired: 13 in]
      }
      frame "---------- New Category ----------" {
        # "Template Separator\n(You can make a copy of, or modify, this frame)"
        n104 = call <vilib>:"Add State(s) to Queue__jki_lib_state_machine.vi"("State(s) in (\"\")"=w231) -> ("States Out"=w230:string)  [unwired: 14 in]
      }
      frame "MakeChart" {
        n105 = Unbundle By Name(w237) -> ("CurrentGraph1"=w239:dbl[][])
        n106 = property on="Current::1" class="DigNum (strict)"() -> ("Value"=w233:dbl)  [unwired: 2 in, 2 out]
        n107 = property on="Current::2" class="DigNum (strict)"() -> ("Value"=w232:dbl)  [unwired: 2 in, 2 out]
        n108 = Build Array(w233, w232) -> (w234:dbl[])
        n109 = Build Array (concatenate)(w239, w234) -> (→"Chart":dbl[][])
      }
    }
  }
